vi "LaserLineDetection_Intensity_incidentAngle.vi"(9 "Camera Parameters":T1, 10 "Distance (D)":dbl, 11 "slope":dbl) -> (2 "Perpendicular Distance (Dp)":dbl, 3 "delta° (incident angle)":dbl)   [LabVIEW 2013]
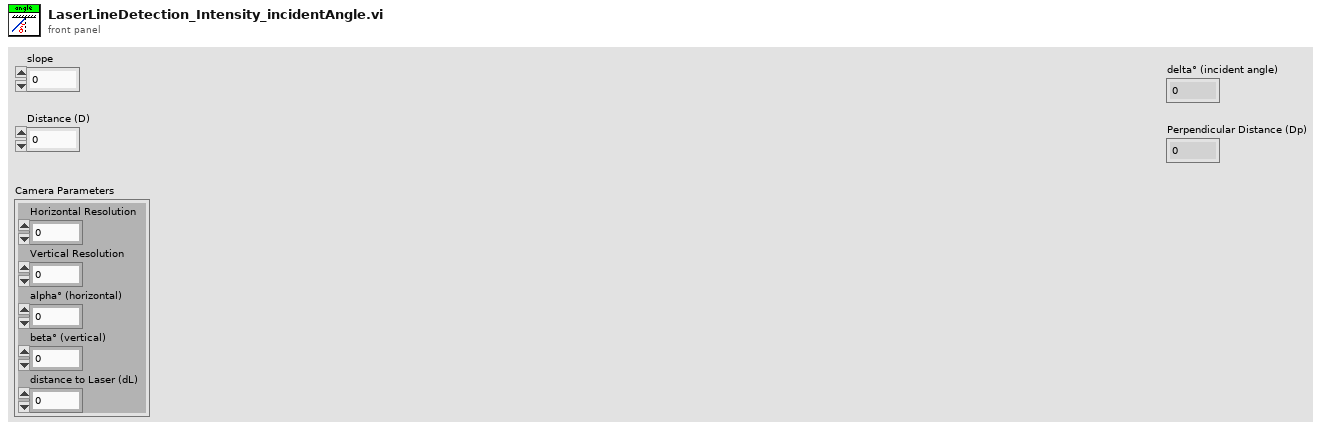
[diagram p1: front panel]
types:
  T1 = cluster{"Horizontal Resolution":dbl, "Vertical Resolution":dbl, "alpha° (horizontal)":dbl, "beta° (vertical)":dbl, "distance to Laser (dL)":dbl}
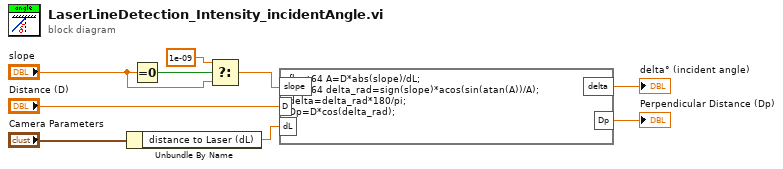
[diagram p0: block diagram]
diagram:
  n1 = Unbundle By Name("Camera Parameters") -> ("distance to Laser (dL)"=w6:dbl)
  n2 = Equal To 0?(x="slope") -> (x = 0?=w4:bool)
  n3 = Select(t=1e-09, s=w4, f="slope") -> (s? t:f=w1:dbl)
  n4 = formula code="float64 A=D*abs(slope)/dL;\nfloat64 delta_rad=sign(slope)*acos(sin(atan(A))/A);\ndelta=delta_rad*180/pi;\nDp=D*cos(delta_rad);"("slope"=w1, "D"="Distance (D)", "dL"=w6) -> ("delta"=→"delta° (incident angle)":dbl, "Dp"=→"Perpendicular Distance (Dp)":dbl)
